vi "Motion manual controls.vi"() -> ()   [LabVIEW 2017]
panel:
  out "Boolean 4":bool
  in  "SetZOrigin 4":bool
  in  "moveToZOrigin 4":bool caption="R Home"
  in  "Position,mm 5":sgl caption="R Position, degrees" format="%.4f"
  in  "Set R Position, mm":sgl format="%.4f"
  in  "Right 4":bool
  in  "Left jog 4":bool
  out "Boolean 3":bool
  in  "SetZOrigin 3":bool
  in  "moveToZOrigin 3":bool caption="Z Home"
  in  "Position,mm 4":sgl caption="Z Position, mm" format="%.4f"
  in  "Set Z Position, mm":sgl format="%.4f"
  in  "Right 3":bool
  in  "Left jog 3":bool
  out "Boolean 2":bool
  in  "SetZOrigin 2":bool
  in  "moveToZOrigin 2":bool caption="Y Home"
  in  "Position,mm 3":sgl caption="Y Position, mm" format="%.4f"
  in  "Set Y Position, mm":sgl format="%.4f"
  in  "Right 2":bool
  in  "Left jog 2":bool
  out "Boolean":bool
  in  "SetZOrigin":bool
  in  "moveToZOrigin":bool caption="X Home"
  in  "Position,mm":sgl caption="X Position, mm" format="%.4f"
  in  "Set X Position, mm":sgl format="%.4f"
  in  "Right":bool
  in  "Left jog":bool
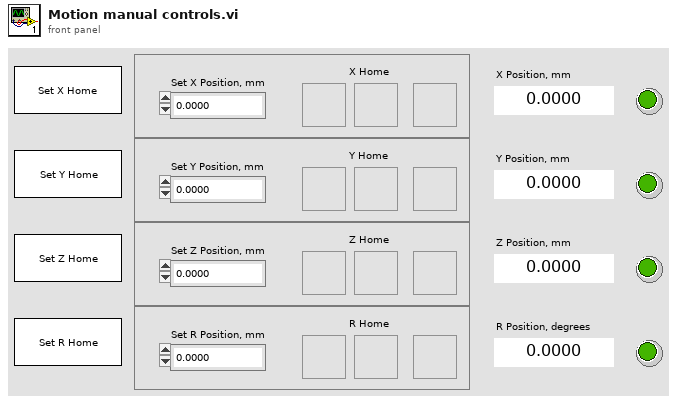
[diagram p1: front panel]
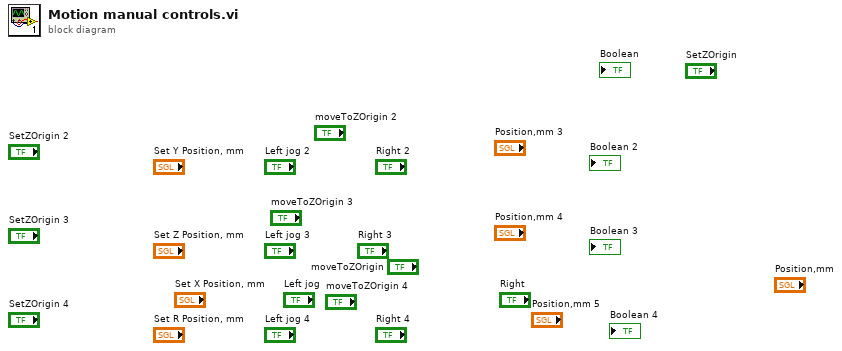
[diagram p0: block diagram]
diagram:
